vi "rescaler.vi"(1 "Min":i32, 2 "Value":i32, 3 "Max":i32) -> (0 "Rescaled value (%)":dbl)   [LabVIEW 2017]
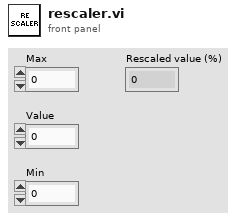
[diagram p1: front panel]
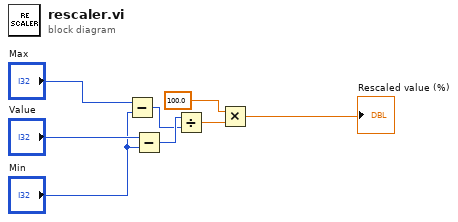
[diagram p0: block diagram]
diagram:
  n1 = Subtract(x="Max", y="Min") -> (x-y=w3:i32)
  n2 = Subtract(x="Value", y="Min") -> (x-y=w4:i32)
  n3 = Divide(x=w4, y=w3) -> (x/y=w2:dbl)
  n4 = Multiply(x=100.0, y=w2) -> (x*y=→"Rescaled value (%)":dbl)
